vi "Run 01.vi"(11 "NXT/EV3 in":T1) -> (3 "EV3 out":T1)   [LabVIEW 2016]
uses:
  <vilib>/NXT/Subs/LVHSConnector.ctl
  <vilib>/NXT/LegoClasses/BrickReference/BrickReference.lvclass
  <vilib>/NXT/Block Support/NXT_ButtonSelector.ctl
  <vilib>/NXT/Dual Mode Library/Waits/Wait_Btn_Press.vi
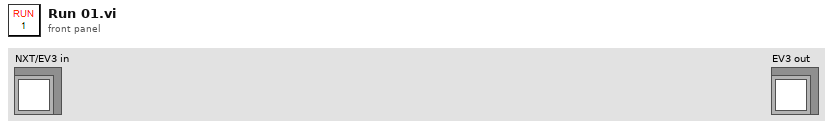
[diagram p1: front panel]
types:
  T1 = typedef "LVHSConnector.ctl" = refnum<class "BrickReference.lvclass">
  T2 = typedef "NXT_ButtonSelector.ctl" = u16
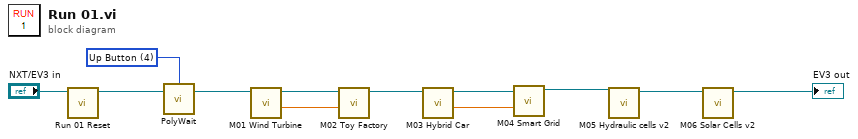
[diagram p0: block diagram]
diagram:
  w6 = T2 4 items=["Enter button"=3, "Left button"=2, "Right button"=1, "Up Button"=4, "Down Button"=5] ("Button (Enter button)")
  n1 = call "Run 01 Reset.vi"("NXT/EV3 in"="NXT/EV3 in") -> ("NXT/EV3 out"=w5:T1)  [unwired: 10 in]
  n2 = call-poly <vilib>:"PolyWait.vi"("NXT/EV3"=w5, "Button (Enter button)"=w6) -> ("NXT/EV3"=w7:T1)  [unwired: 2 in]
  n3 = call "M01 Wind Turbine.vi"("NXT/EV3"=w7) -> ("Angle out"=w11:sgl, "EV3 out"=w12:T1)  [unwired: 9 in]
  n4 = call "M02 Toy Factory.vi"("Angle in"=w11, "EV3 in"=w12) -> ("EV3 out"=w10:T1)  [unwired: 9 in]
  n5 = call "M03 Hybrid Car.vi"("EV3 in"=w10) -> ("Angle out"=w8:sgl, "EV3 out"=w9:T1)  [unwired: 9 in]
  n6 = call "M04 Smart Grid.vi"("Target angle"=w8, "EV3 in"=w9) -> ("EV3 out"=w4:T1)  [unwired: 9 in]
  n7 = call "M05 Hydraulic cells v2.vi"("EV3 in"=w4) -> ("EV3 out"=w3:T1)  [unwired: 10 in]
  n8 = call "M06 Solar Cells v2.vi"("EV3 in"=w3) -> ("EV3 out"=→"EV3 out":T1)  [unwired: 10 in]
